vi "Find Module In Project and Open Main.vi"(8 "error in":errorcluster, 10 "Library in":refnum<class "Library.lvclass">, 11 "Project":refnum<class "Project.lvclass">) -> (0 "error out":errorcluster, 3 "Project out":refnum<class "Project.lvclass">)   [LabVIEW 2020, in "Panther Dashboard.lvlib"]
uses:
  Panther Dashboard.lvlib
  Class/Project/Project.lvclass
  Class/Library/Library.lvclass
  C:/GitClones/PantherDashboard/src/LabVIEW/Panther Dashboard/Class/LabVIEWItem/LabVIEWItem.lvclass
  Class/Project/Project.lvclass/Project.ctl
  Class/Library/Library.lvclass/Library.ctl
  Class/LabVIEWItem/LabVIEWItem.lvclass/LabVIEWItem.ctl
  Class/Project/Read Project Ref.vi
  Class/Project/Read Main App Inst Ref.vi
  Class/Library/Read Dependency.vi
  Class/Library/Read Library Ref.vi
  Class/LabVIEWItem/Read Item Path.vi
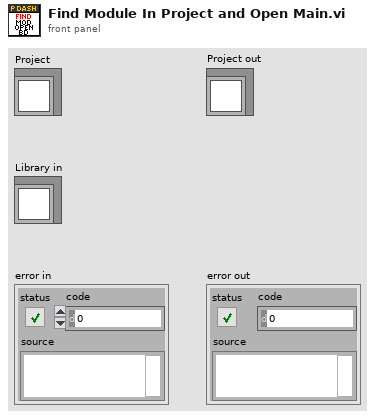
[diagram p1: front panel]
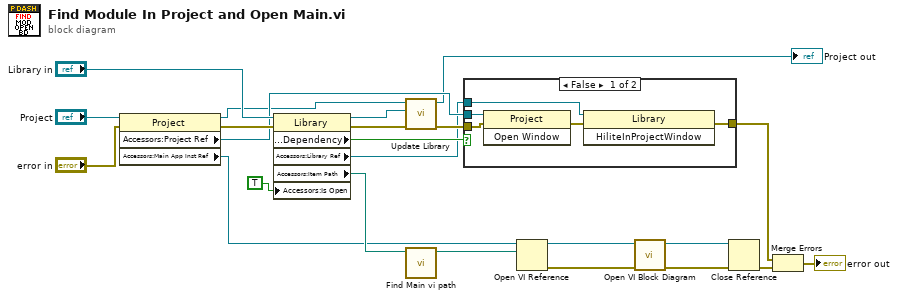
[diagram p0: block diagram]
diagram:
  n1 = property class="Project"(reference="Project", error in="error in") -> (reference out=w3:refnum<class "Project.lvclass">, error out=w17:errorcluster, "Accessors:Project Ref"=w7:refnum<vi>, "Accessors:Main App Inst Ref"=w8:refnum<vi>)
  n2 = property class="Library"(reference="Library in", error in=w17, "Accessors:Is Open"=TRUE ("Is Open")) -> (reference out=w2:refnum<class "Library.lvclass">, error out=w16:errorcluster, "Accessors:Dependency"=w6:bool, "Accessors:Library Ref"=w5:refnum<vi>, "Accessors:Item Path"=w14:path)
  n3 = call "Update Library.vi"("error in"=w16, "Library"=w2, "Project in"=w3) -> ("error out"=w15:errorcluster, "Project out"=→"Project out":refnum<class "Project.lvclass">)  [unwired: 7 in]
  n4 = call "Find Main vi path.vi"("Library Path"=w14) -> ("Main vi Path"=w11:path)  [unwired: 8 in, 2 out]
  n5 = case shown="False" w6 {
    tunnel: [w28 w29] -> w23
    tunnel: w7 -> [w25 _]
    tunnel: w15 -> [w27 w29]
    tunnel: w5 -> [w24 _]
    frame False {
      n6 = invoke class="Project" method="Open Window"(reference=w25, error in=w27) -> (error out=w26:errorcluster)  [unwired: 1 in, 2 out]
      n7 = invoke class="Library" method="HiliteInProjectWindow"(reference=w24, error in=w26) -> (error out=w28:errorcluster)  [unwired: 1 in, 2 out]
    }
    frame True {
    }
  }
  n8 = Open VI Reference(application reference (local)=w8, vi path=w11) -> (vi reference=w10:refnum<vi>, error out=w21:errorcluster)  [unwired: 4 in]
  n9 = call "Open VI Block Diagram.vi"("error in"=w21, "VI in"=w10) -> ("error out"=w20:errorcluster, "VI out"=w9:refnum<vi>)  [unwired: 8 in]
  n10 = Close Reference(reference=w9, error in (no error)=w20) -> (error out=w18:errorcluster)
  n11 = Merge Errors(w23, w18) -> (→"error out":errorcluster)
